vi "ti_bridge_temperature.vi"(2 "Z":cdb[][](array[numeric])=[[24.0+0.0i, 231.0+3.0i, 1.0-1.0i, 3.0+2.0i], [43.0+5.0i, 1.0+24.0i, 11.0+0.0i, 0.0+9.0i], [8.0+0.0i, 231.0+0.0i, 231.0+0.0i, 231.0+0.0i], [5.0+0.0i, 0.0+9.0i, 231.0+0.0i, 0.0-3.0i]], 3 "Temperature":dbl[](array[numeric])) -> (0 "Z_array sorted":cdb[][](array[numeric]), 1 "Temperature sorted":dbl[](array[numeric]))   [LabVIEW 2013]
uses:
  vs_bridge/Debug/vs_bridge.dll
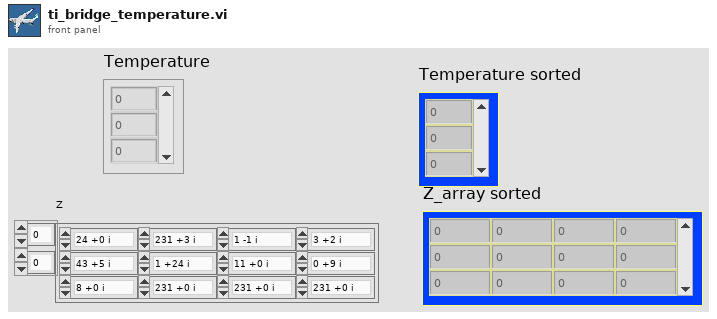
[diagram p1: front panel]
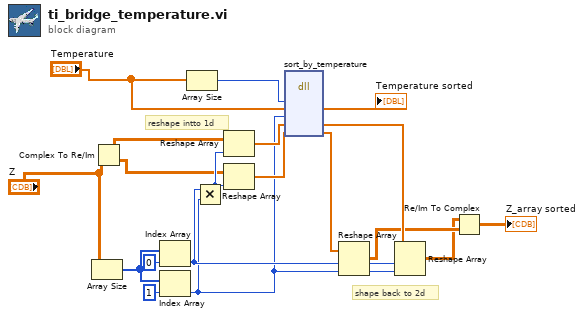
[diagram p0: block diagram]
diagram:
  # "shape back to 2d"
  # "reshape intto 1d"
  n1 = Array Size(array="Z") -> (size(s)=w16:i32[])
  n2 = Complex To Re/Im(x + iy="Z") -> (x=w13:dbl[][], y=w7:dbl[][])
  n3 = Index Array(array=w16, index=0) -> (element=w5:i32)
  n4 = Index Array(array=w16, index=1) -> (element=w4:i32)
  n5 = Array Size(array="Temperature") -> (size(s)=w19:i32)
  n6 = Multiply(x=w5, y=w4) -> (x*y=w14:i32)
  n7 = Reshape Array(w13, w14) -> (w12:dbl[])
  n8 = Reshape Array(w7, w14) -> (w11:dbl[])
  n9 = dll-call lib="C:/Users/astafiev/Desktop/IlyaDrive/@photonCounting/@Programs/ti_bridge/vs_bridge/Debug/vs_bridge.dll" fn="sort_by_temperature"("no_temperatures"=w19, "array_temperature"="Temperature", "readings_per_temperature"=w4, "array_re"=w12, "array_im"=w11) -> ("array_temperature"=→"Temperature sorted":dbl[], "array_re"=w8:dbl[], "array_im"=w6:dbl[])  [unwired: 6 in, 2 out]
  n10 = Reshape Array(w6, w5, w4) -> (w2:dbl[][])
  n11 = Reshape Array(w8, w5, w4) -> (w1:dbl[][])
  n12 = Re/Im To Complex(1:w2, 2:w1) -> (0:→"Z_array sorted":cdb[][])
